vi "Calibration Table.vi"() -> ()   [LabVIEW 2015]
uses:
  Type/_RT Command.ctl
  Type/_File Type.ctl
  <vilib>/Utility/config.llb/Read Key (String).vi
  Configuration/_Global Configuration.vi
  <vilib>/Utility/config.llb/Write Key (String).vi
  <vilib>/Utility/file.llb/Read From Spreadsheet File (DBL).vi
  <vilib>/Utility/config.llb/NI_LVConfig.lvlib
panel:
  in  "Export":bool
  in  "Import":bool
  in  "TableFiles":path[](array[path])=[path "C:/Documents and Settings/MYANG/My Documents/Ion Sniffer/Build/Default Q1 Calibration.cal", path "C:/Documents and Settings/MYANG/My Documents/Ion Sniffer/Build/Default Q2 Calibration.cal", path "C:/Documents and Settings/MYANG/My Documents/Ion Sniffer/Build/Default Q1 Calibration.cal", path "C:/Documents and Settings/MYANG/My Documents/Ion Sniffer/Build/Default Q2 Calibration.cal", path "C:/Documents and Settings/MYANG/My Documents/Ion Sniffer/Build/Default Q1 Resolution.res", path "C:/Documents and Settings/MYANG/My Documents/Ion Sniffer/Build/Default Q2 Resolution.res", path "C:/Documents and Settings/MYANG/My Documents/Ion Sniffer/Build/Default Q1 Resolution.res", path "C:/Documents and Settings/MYANG/My Documents/Ion Sniffer/Build/Default Q2 Resolution.res", path "C:/Documents and Settings/MYANG/My Documents/Ion Sniffer/Build/Default Q1 Resolution.res", path "C:/Documents and Settings/MYANG/My Documents/Ion Sniffer/Build/Default Q2 Resolution.res", path "C:/Documents and Settings/MYANG/My Documents/Ion Sniffer/Build/Default Q1 Resolution.res", path "C:/Documents and Settings/MYANG/My Documents/Ion Sniffer/Build/Default Q2 Resolution.res", path "C:/Documents and Settings/MYANG/My Documents/Ion Sniffer/Build/Default Q1 Resolution.res", path "C:/Documents and Settings/MYANG/My Documents/Ion Sniffer/Build/Default Q2 Resolution.res", path "C:/Documents and Settings/MYANG/My Documents/Ion Sniffer/Build/Default Q1 Resolution.res", path "C:/Documents and Settings/MYANG/My Documents/Ion Sniffer/Build/Default Q2 Resolution.res"]
  in  "Measured Mass":dbl=50.0 caption="Measured Mass\n(amu)" min=0.0 format="%#.6g"
  in  "Reference Mass":dbl=50.0 caption="Reference Mass\n(amu)" min=0.0 format="%#.6g"
  in  "DAC Value":i32=8340 min=0 step=1
  in  "Download":bool
  in  "UITable":i32(listbox)
  in  "Table Type":u16(ring) items=["Q1 +ve Mass Calibration Table", "Q2 +ve Mass Calibration Table", "Q1 -ve Mass Calibration Table", "Q2 -ve Mass Calibration Table", "Q1 +ve High Resolution Table", "Q2 +ve High Resolution Table", "Q1 +ve Medium Resolution Table", "Q2 +ve Medium Resolution Table", "Q1 +ve Low Resolution Table", "Q2 +ve Low Resolution Table", "Q1 -ve High Resolution Table", "Q2 -ve High Resolution Table", "Q1 -ve Medium Resolution Table", "Q2 -ve Medium Resolution Table", "Q1 -ve Low Resolution Table", "Q2 -ve Low Resolution Table"]
  in  "Change":bool
  in  "Current Point #:":i32=1 min=1 step=1
  in  "Delete":bool
  in  "Insert":bool
  out "File Path:":path=path "C:/Documents and Settings/MYANG/My Documents/Ion Sniffer/Build/Default Q2 Resolution.res"
  in  "Save":bool
  in  "Load":bool
  out "Graph":cluster{"all rows":dbl[], "all rows":dbl[]}(graph)={"all rows"=[50.0, 130.0, 174.0, 195.0, 397.0, 510.0, 609.0, 906.0], "all rows"=[8340.0, 8620.0, 8730.0, 8825.0, 9480.0, 9830.0, 10230.0, 11000.0]} caption="Q1 Mass Calibration"
  out "# of Entries":i32=8
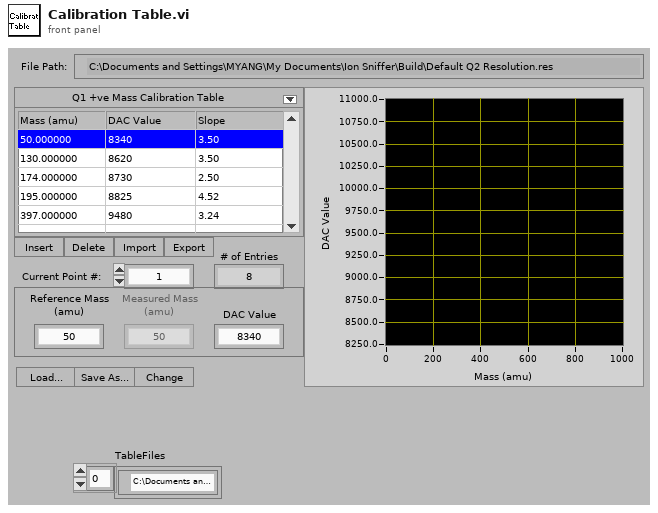
[diagram p1: front panel]
types:
  T1 = typedef "_RT Command.ctl" = enum16{"Start", "StartActualRun", "Stop", "Runtime Update", "Get Data", "Get Info", "Get Status", "Get Param", "Get Config", "Get Table", "Read ADC", "Set Oscillator", "Update Config", "Update Table", "Set All Pol", "Set Pol and DC", "Set Max Mass", "Toggle RP", "Toggle EL", "Set PIC", "Initialize Turbo", "Send Turbo Comm", "Close Turbo", "P1", "P2", "P3", "Send Serial", "Set LC Out", "Get LC In", "Read VAC", "Test Table", "Toggle Power", "Get Startup", "Set Startup", "Get ADC Table", "Set ADC Table", "Get Brief Status", "Get Detail Status", "Auxiliary Update", "Set CC Logics", "Set CC Input Logics", "Ignore Error"}
  T2 = typedef "_File Type.ctl" = enum16{"Configuration", "Old Configuration", "Calibration", "Resolution", "Diagnostic Method", "Old Method", "Acq Method", "Samp List"}
  T3 = enum32{"existing file", "new file", "new or existing file", "existing dir", "new dir", "new or existing dir", "existing file (use LLBs)", "new file (use LLBs)", "new or existing file (use LLBs)", "new or existing file or directory (use LLBs)"}
  T4 = typedef "NI_LVConfig.lvlib/Config Data RefNum.ctl" = refnum<k1>
  T5 = cluster{"Table":dbl[][], "Current Point #:":i32, "Update":bool, "TableFiles":path[]}
  T6 = typedef "_RT Configuration 2.ctl" = cluster{"Name":string, "Ch#":u8, "Min":dbl, "Max":dbl, "Def+":dbl, "Def-":dbl, "Offset":dbl, "Slope":dbl, "Type":u8, "Description":string, "SettleT":dbl}
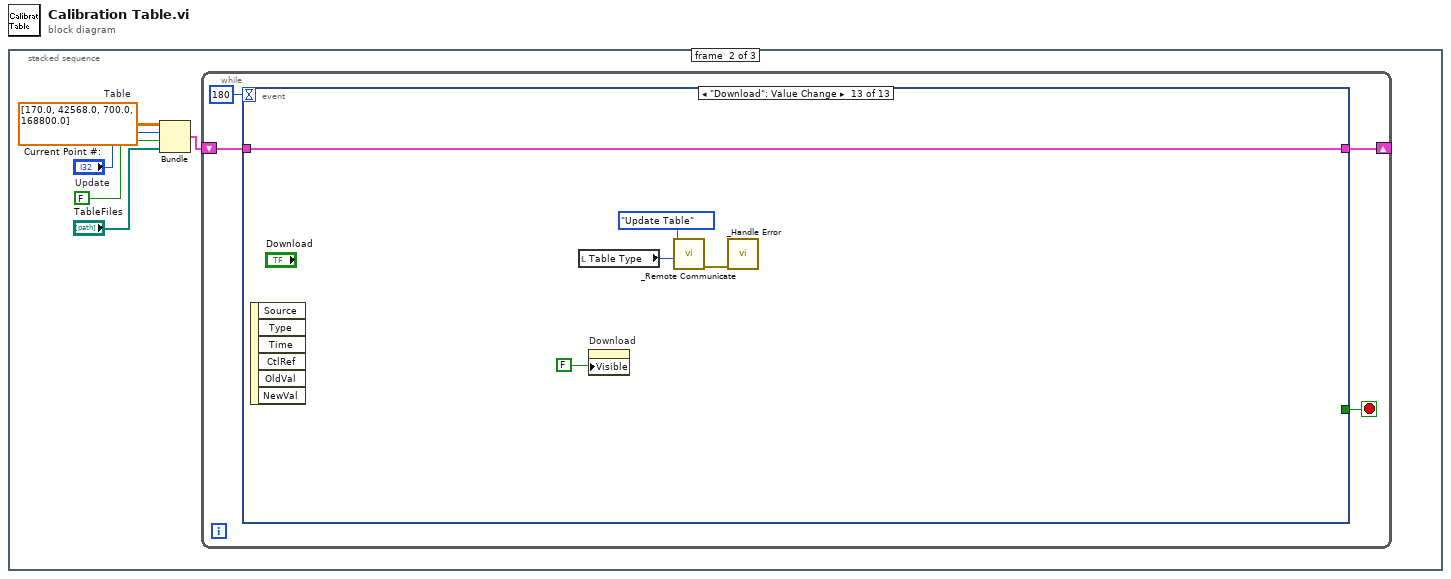
[diagram p0: block diagram]
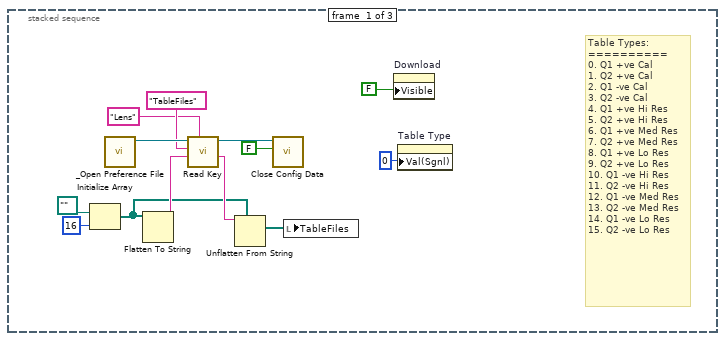
[diagram p2: hidden frame]
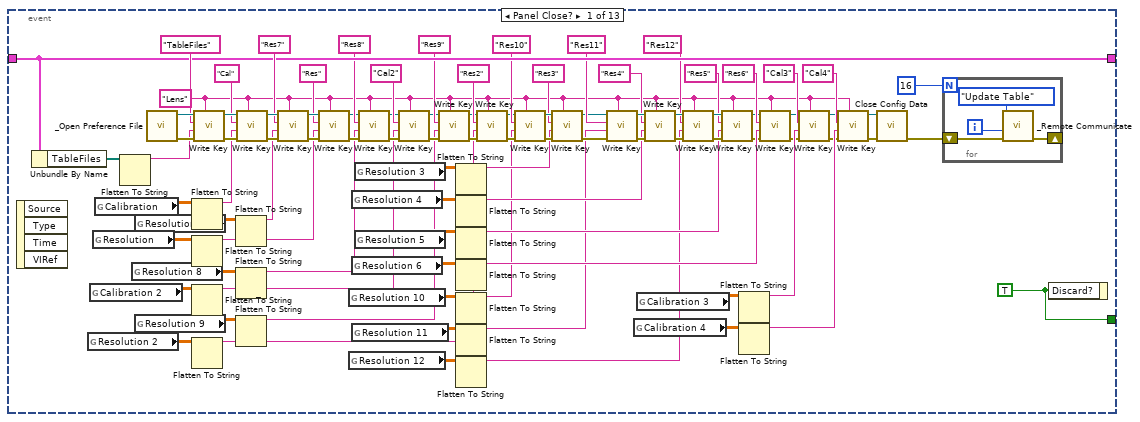
[diagram p3: hidden frame]
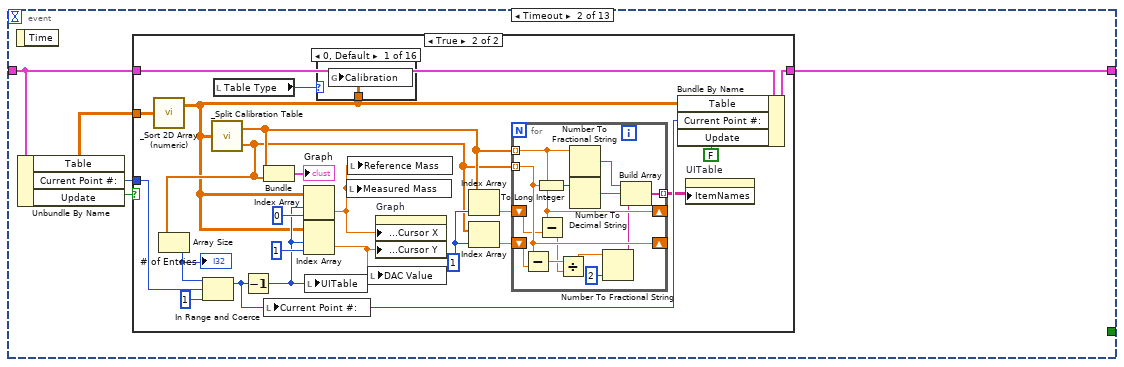
[diagram p4: hidden frame]
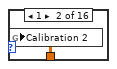
[diagram p6: hidden frame]
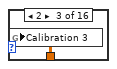
[diagram p7: hidden frame]
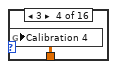
[diagram p8: hidden frame]
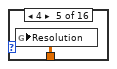
[diagram p9: hidden frame]
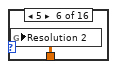
[diagram p10: hidden frame]
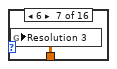
[diagram p11: hidden frame]
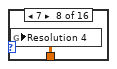
[diagram p12: hidden frame]
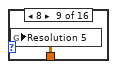
[diagram p13: hidden frame]
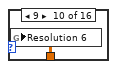
[diagram p14: hidden frame]
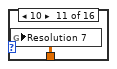
[diagram p15: hidden frame]
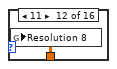
[diagram p16: hidden frame]
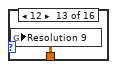
[diagram p17: hidden frame]
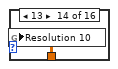
[diagram p18: hidden frame]
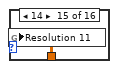
[diagram p19: hidden frame]
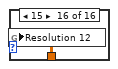
[diagram p20: hidden frame]
diagram:
  n1 = stacked-sequence {
    frame #0 {
      # "Table Types:\n==========\n0. Q1 +ve Cal\n1. Q2 +ve Cal\n2. Q1 -ve Cal\n3. Q2 -ve Cal\n4. Q1 +ve Hi Res\n5. Q2 +ve Hi Res\n6. Q1 +ve Med Res\n7. Q2 +ve Med Res\n8. Q1 +ve Lo Res\n9. Q2 +ve Lo Res\n10. Q1 -ve Hi Res\n11. Q2 -ve Hi Res\n12. Q1 -ve Med Res\n13. Q2 -ve Med Res\n14. Q1 -ve Lo Res\n15. Q2 -ve Lo Res"
      n2 = Initialize Array(path "", 16 ("dimension size")) -> (w2:path[])
      n3 = call "_Open Preference File.vi"() -> ("refnum"=w13:T4)  [unwired: 2 in, 5 out]
      n4 = Flatten To String(anything=w2) -> (data string=w7:string)  [unwired: 1 in, 4 out]
      n5 = call-poly <vilib>:"Read Key.vi"("section"="Lens", "default value"=w7, "key"="TableFiles" ("section"), "refnum"=w13) -> ("value"=w6:string, "refnum out"=w5:T4)  [unwired: 2 in, 4 out]
      n6 = Unflatten From String(type=w2, binary string=w6) -> (value=w1:path[])  [unwired: 1 in, 4 out]
      n7 = call <vilib>:"Close Config Data.vi"("write file if changed (T)"=FALSE ("write configuration file? (T)"), "refnum"=w5) -> ()  [unwired: 1 in, 9 out]
      n8 = local write "TableFiles"(w1) -> ()
      n9 = property on="Download" class="Bool"("Visible"=FALSE) -> ()  [unwired: 2 in, 2 out]
      n10 = property on="Table Type" class="Ring (strict)"("Val(Sgnl)"=u16 0 ("Value (Signaling)")) -> ()  [unwired: 2 in, 2 out]
    }
    frame #1 {
      w17 = FALSE  # Update
      w18 = dbl[][] [[170.0, 42568.0], [700.0, 168800.0]]  # Table
      n11 = Bundle("Table"=w18, "Current Point #:"="Current Point #:", "Update"=w17, "TableFiles"="TableFiles") -> (w16:T5)  [unwired: 1 out]
      n12 = while {
        shift-right: [w20] -> _
        shift-left: w16 -> [w21]
        stop <- w19 stop-if-true
        n13 = event shown="[12] \"Download\": Value Change" {
          selector: _ -> [_ _ _ _ _ _ _ _ _ _ _ _ _]
          dyn-events: _ -> [_ _ _ _ _ _ _ _ _ _ _ _ _]
          timeout: 180 -> [_ _ _ _ _ _ _ _ _ _ _ _ _]
          tunnel: w21 -> [w97 w121 w181 w238 w242 w246 w267 w287 w307 w333 w390 w416 w431]
          tunnel: [w97 w120 w185 w237 w241 w245 w266 w294 w307 w332 w389 w415 w431] -> w20
          tunnel: [w114 _ _ _ _ _ _ _ _ _ _ _ _] -> w19
          event Panel Close? {
            w51 = "Lens" ("section")
            w114 = TRUE ("Discard?")
            n14 = event-data() -> ()  [unwired: 5 out]
            n15 = Unbundle By Name(w97) -> ("TableFiles"=w44:path[])
            n16 = global read "_Global Configuration.vi" "Resolution 2"() -> (w84:dbl[][])
            n17 = global read "_Global Configuration.vi" "Calibration 2"() -> (w83:dbl[][])
            n18 = global read "_Global Configuration.vi" "Resolution"() -> (w99:dbl[][])
            n19 = global read "_Global Configuration.vi" "Calibration"() -> (w101:dbl[][])
            n20 = Flatten To String(anything=w44) -> (data string=w43:string)  [unwired: 1 in, 4 out]
            n21 = global read "_Global Configuration.vi" "Resolution 8"() -> (w38:dbl[][])
            n22 = global read "_Global Configuration.vi" "Resolution 7"() -> (w37:dbl[][])
            n23 = global read "_Global Configuration.vi" "Resolution 9"() -> (w39:dbl[][])
            n24 = call "_Open Preference File.vi"() -> ("error"=w110:errorcluster, "refnum"=w111:T4)  [unwired: 2 in, 4 out]
            n25 = Flatten To String(anything=w101) -> (data string=w100:string)  [unwired: 1 in, 4 out]
            n26 = Flatten To String(anything=w99) -> (data string=w98:string)  [unwired: 1 in, 4 out]
            n27 = Flatten To String(anything=w83) -> (data string=w82:string)  [unwired: 1 in, 4 out]
            n28 = Flatten To String(anything=w84) -> (data string=w81:string)  [unwired: 1 in, 4 out]
            n29 = call-poly <vilib>:"Write Key.vi"("section"=w51, "error in (no error)"=w110, "value"=w43, "key"="TableFiles" ("section"), "refnum"=w111) -> ("error out"=w113:errorcluster, "refnum out"=w112:T4)  [unwired: 1 in, 4 out]
            n30 = Flatten To String(anything=w37) -> (data string=w36:string)  [unwired: 1 in, 4 out]
            n31 = Flatten To String(anything=w38) -> (data string=w35:string)  [unwired: 1 in, 4 out]
            n32 = Flatten To String(anything=w39) -> (data string=w34:string)  [unwired: 1 in, 4 out]
            n33 = call-poly <vilib>:"Write Key.vi"("section"=w51, "error in (no error)"=w113, "value"=w100, "key"="Cal" ("section"), "refnum"=w112) -> ("error out"=w107:errorcluster, "refnum out"=w106:T4)  [unwired: 1 in, 4 out]
            n34 = call-poly <vilib>:"Write Key.vi"("section"=w51, "error in (no error)"=w107, "value"=w36, "key"="Res7" ("section"), "refnum"=w106) -> ("error out"=w108:errorcluster, "refnum out"=w109:T4)  [unwired: 1 in, 4 out]
            n35 = call-poly <vilib>:"Write Key.vi"("section"=w51, "error in (no error)"=w108, "value"=w98, "key"="Res" ("section"), "refnum"=w109) -> ("error out"=w86:errorcluster, "refnum out"=w85:T4)  [unwired: 1 in, 4 out]
            n36 = global read "_Global Configuration.vi" "Resolution 10"() -> (w33:dbl[][])
            n37 = global read "_Global Configuration.vi" "Resolution 12"() -> (w32:dbl[][])
            n38 = global read "_Global Configuration.vi" "Resolution 4"() -> (w59:dbl[][])
            n39 = global read "_Global Configuration.vi" "Resolution 6"() -> (w60:dbl[][])
            n40 = global read "_Global Configuration.vi" "Resolution 11"() -> (w31:dbl[][])
            n41 = global read "_Global Configuration.vi" "Resolution 3"() -> (w58:dbl[][])
            n42 = global read "_Global Configuration.vi" "Resolution 5"() -> (w61:dbl[][])
            n43 = call-poly <vilib>:"Write Key.vi"("section"=w51, "error in (no error)"=w86, "value"=w35, "key"="Res8" ("section"), "refnum"=w85) -> ("error out"=w87:errorcluster, "refnum out"=w88:T4)  [unwired: 1 in, 4 out]
            n44 = call-poly <vilib>:"Write Key.vi"("section"=w51, "error in (no error)"=w87, "value"=w82, "key"="Cal2" ("section"), "refnum"=w88) -> ("error out"=w91:errorcluster, "refnum out"=w92:T4)  [unwired: 1 in, 4 out]
            n45 = call-poly <vilib>:"Write Key.vi"("section"=w51, "error in (no error)"=w91, "value"=w34, "key"="Res9" ("section"), "refnum"=w92) -> ("error out"=w90:errorcluster, "refnum out"=w89:T4)  [unwired: 1 in, 4 out]
            n46 = Flatten To String(anything=w58) -> (data string=w57:string)  [unwired: 1 in, 4 out]
            n47 = Flatten To String(anything=w59) -> (data string=w56:string)  [unwired: 1 in, 4 out]
            n48 = Flatten To String(anything=w61) -> (data string=w55:string)  [unwired: 1 in, 4 out]
            n49 = Flatten To String(anything=w60) -> (data string=w54:string)  [unwired: 1 in, 4 out]
            n50 = Flatten To String(anything=w33) -> (data string=w30:string)  [unwired: 1 in, 4 out]
            n51 = Flatten To String(anything=w31) -> (data string=w29:string)  [unwired: 1 in, 4 out]
            n52 = Flatten To String(anything=w32) -> (data string=w28:string)  [unwired: 1 in, 4 out]
            n53 = call-poly <vilib>:"Write Key.vi"("section"=w51, "error in (no error)"=w90, "value"=w81, "key"="Res2" ("section"), "refnum"=w89) -> ("error out"=w75:errorcluster, "refnum out"=w76:T4)  [unwired: 1 in, 4 out]
            n54 = call-poly <vilib>:"Write Key.vi"("section"=w51, "error in (no error)"=w75, "value"=w30, "key"="Res10" ("section"), "refnum"=w76) -> ("error out"=w79:errorcluster, "refnum out"=w80:T4)  [unwired: 1 in, 4 out]
            n55 = call-poly <vilib>:"Write Key.vi"("section"=w51, "error in (no error)"=w79, "value"=w57, "key"="Res3" ("section"), "refnum"=w80) -> ("error out"=w63:errorcluster, "refnum out"=w62:T4)  [unwired: 1 in, 4 out]
            n56 = call-poly <vilib>:"Write Key.vi"("section"=w51, "error in (no error)"=w63, "value"=w29, "key"="Res11" ("section"), "refnum"=w62) -> ("error out"=w73:errorcluster, "refnum out"=w72:T4)  [unwired: 1 in, 4 out]
            n57 = global read "_Global Configuration.vi" "Calibration 4"() -> (w50:dbl[][])
            n58 = global read "_Global Configuration.vi" "Calibration 3"() -> (w49:dbl[][])
            n59 = call-poly <vilib>:"Write Key.vi"("section"=w51, "error in (no error)"=w73, "value"=w56, "key"="Res4" ("section"), "refnum"=w72) -> ("error out"=w69:errorcluster, "refnum out"=w68:T4)  [unwired: 1 in, 4 out]
            n60 = call-poly <vilib>:"Write Key.vi"("section"=w51, "error in (no error)"=w69, "value"=w28, "key"="Res12" ("section"), "refnum"=w68) -> ("error out"=w70:errorcluster, "refnum out"=w71:T4)  [unwired: 1 in, 4 out]
            n61 = call-poly <vilib>:"Write Key.vi"("section"=w51, "error in (no error)"=w70, "value"=w55, "key"="Res5" ("section"), "refnum"=w71) -> ("error out"=w27:errorcluster, "refnum out"=w42:T4)  [unwired: 1 in, 4 out]
            n62 = Flatten To String(anything=w49) -> (data string=w48:string)  [unwired: 1 in, 4 out]
            n63 = Flatten To String(anything=w50) -> (data string=w47:string)  [unwired: 1 in, 4 out]
            n64 = call-poly <vilib>:"Write Key.vi"("section"=w51, "error in (no error)"=w27, "value"=w54, "key"="Res6" ("section"), "refnum"=w42) -> ("error out"=w26:errorcluster, "refnum out"=w41:T4)  [unwired: 1 in, 4 out]
            n65 = call-poly <vilib>:"Write Key.vi"("section"=w51, "error in (no error)"=w26, "value"=w48, "key"="Cal3" ("section"), "refnum"=w41) -> ("error out"=w25:errorcluster, "refnum out"=w40:T4)  [unwired: 1 in, 4 out]
            n66 = call-poly <vilib>:"Write Key.vi"("section"=w51, "error in (no error)"=w25, "value"=w47, "key"="Cal4" ("section"), "refnum"=w40) -> ("error out"=w45:errorcluster, "refnum out"=w46:T4)  [unwired: 1 in, 4 out]
            n67 = call <vilib>:"Close Config Data.vi"("error in (no error)"=w45, "refnum"=w46) -> ("error out"=w24:errorcluster)  [unwired: 1 in, 8 out]
            n68 = for {
              N: 16 -> [_]
              shift-right: [w116] -> _
              shift-left: w24 -> [w117]
              i -> [w115]
              n69 = call "_Remote Communicate.vi"("error in (no error)"=w117, "DC Param"=w115, "Command"=_RT_Command."Update Table") -> ("error out"=w116:errorcluster)  [unwired: 3 in, 3 out]
            }
            n70 = event-data("Discard?"=w114) -> ()  [unwired: 1 in, 1 out]
          }
          event Timeout {
            n71 = event-data() -> ()  [unwired: 2 out]
            n72 = Unbundle By Name(w121) -> ("Table"=w119:dbl[][], "Current Point #:"=w122:i32, "Update"=w123:bool)
            n73 = case shown="True" w123 {
              tunnel: w119 -> [_ w141]
              tunnel: w122 -> [_ w143]
              tunnel: w121 -> [w124 w140]
              tunnel: [w124 w139] -> w120
              frame False {
              }
              frame True {
                w131 = 1 ("index")
                n74 = call "_Sort 2D Array (numeric).vi"("Unsorted 2D Array"=w141) -> ("Sorted 2D Array"=w126:dbl[][])  [unwired: 4 in, 1 out]
                n75 = call "_Split Calibration Table.vi"("Calibration"=w126) -> ("Mass"=w132:dbl[], "DAC"=w130:dbl[])
                n76 = Array Size(array=w130) -> (size(s)=w134:i32)
                "# of Entries" <- w134
                n77 = In Range and Coerce(upper limit=w134, x=w143, lower limit=1) -> (coerced(x)=w138:i32)  [unwired: 1 out]
                n78 = local read "Table Type"() -> (w127:u16)
                n79 = Decrement(x=w138) -> (x-1=w142:i32)
                n80 = Bundle("Mass"=w132, "DAC"=w130) -> (→"Graph":cluster{"Mass":dbl[], "DAC":dbl[]})  [unwired: 1 out]
                n81 = local write "Current Point #:"(w138) -> ()
                n82 = Index Array(array=w126, index (row)=w142, index (col)=0 ("Index")) -> (element=w135:dbl)
                n83 = Index Array(array=w126, index (row)=w142, index (col)=1 ("Index")) -> (element=w125:dbl)
                n84 = local write "UITable"(w142) -> ()
                n85 = case shown="0, Default" w127 {
                  tunnel: w126 -> [w147 w148 w149 w150 w151 w152 w153 w154 w155 w156 w157 w158 w159 w160 w161 w162]
                  frame 0, Default {
                    n86 = global write "_Global Configuration.vi" "Calibration"(w147) -> ()
                  }
                  frame 1 {
                    n87 = global write "_Global Configuration.vi" "Calibration 2"(w148) -> ()
                  }
                  frame 2 {
                    n88 = global write "_Global Configuration.vi" "Calibration 3"(w149) -> ()
                  }
                  frame 3 {
                    n89 = global write "_Global Configuration.vi" "Calibration 4"(w150) -> ()
                  }
                  frame 4 {
                    n90 = global write "_Global Configuration.vi" "Resolution"(w151) -> ()
                  }
                  frame 5 {
                    n91 = global write "_Global Configuration.vi" "Resolution 2"(w152) -> ()
                  }
                  frame 6 {
                    n92 = global write "_Global Configuration.vi" "Resolution 3"(w153) -> ()
                  }
                  frame 7 {
                    n93 = global write "_Global Configuration.vi" "Resolution 4"(w154) -> ()
                  }
                  frame 8 {
                    n94 = global write "_Global Configuration.vi" "Resolution 5"(w155) -> ()
                  }
                  frame 9 {
                    n95 = global write "_Global Configuration.vi" "Resolution 6"(w156) -> ()
                  }
                  frame 10 {
                    n96 = global write "_Global Configuration.vi" "Resolution 7"(w157) -> ()
                  }
                  frame 11 {
                    n97 = global write "_Global Configuration.vi" "Resolution 8"(w158) -> ()
                  }
                  frame 12 {
                    n98 = global write "_Global Configuration.vi" "Resolution 9"(w159) -> ()
                  }
                  frame 13 {
                    n99 = global write "_Global Configuration.vi" "Resolution 10"(w160) -> ()
                  }
                  frame 14 {
                    n100 = global write "_Global Configuration.vi" "Resolution 11"(w161) -> ()
                  }
                  frame 15 {
                    n101 = global write "_Global Configuration.vi" "Resolution 12"(w162) -> ()
                  }
                }
                n102 = local write "Measured Mass"(w135) -> ()
                n103 = local write "Reference Mass"(w135) -> ()
                n104 = local write "DAC Value"(w125) -> ()
                n105 = property on="Graph" class="XYGraph (strict)"("Cursor.Cursor Position:Cursor X"=w135, "Cursor.Cursor Position:Cursor Y"=w125) -> ()  [unwired: 2 in, 2 out]
                n106 = Index Array(array=w132, index=w131) -> (element=w129:dbl)
                n107 = Index Array(array=w130, index=w131) -> (element=w128:dbl)
                n108 = for {
                  tunnel: [w172] -> w133 mode=indexing
                  tunnel: w132 -> [w169] mode=indexing
                  tunnel: w130 -> [w171] mode=indexing
                  shift-right: [w169] -> _
                  shift-left: w129 -> [w168]
                  shift-right: [w171] -> _
                  shift-left: w128 -> [w170]
                  n109 = Subtract(x=w171, y=w170) -> (x-y=w167:dbl)
                  n110 = To Long Integer(number=w171) -> (32bit integer=w175:i32)
                  n111 = Subtract(x=w169, y=w168) -> (x-y=w166:dbl)
                  n112 = Divide(x=w167, y=w166) -> (x/y=w165:dbl)
                  n113 = Number To Fractional String(number=w169) -> (F-format string=w174:string)  [unwired: 3 out]
                  n114 = Number To Decimal String(number=w175) -> (decimal integer string=w173:string)  [unwired: 1 out]
                  n115 = Number To Fractional String(number=w165, precision (6)=i16 2) -> (F-format string=w163:string)  [unwired: 2 out]
                  n116 = Build Array(w174, w173, w163) -> (w172:string[])
                }
                n117 = Bundle By Name(cluster=w140, "Table"=w126, "Current Point #:"=w138, "Update"=FALSE) -> (w139:T5)
                n118 = property on="UITable" class="MCListbox (strict)"("ItemNames"=w133) -> ()  [unwired: 2 in, 2 out]
              }
            }
          }
          event "Table Type": Value Change {
            n119 = event-data() -> ("NewVal"=w177:u16)  [unwired: 1 out]
            n120 = Unbundle By Name(w181) -> ("TableFiles"=w178:path[])
            n121 = Index Array(array=w178, index=w177) -> (element=w176:path)
            n122 = local write "File Path:"(w176) -> ()
            n123 = case shown="0, Default" w177 {
              tunnel: [w188 w191 w194 w197 w200 w203 w206 w209 w212 w215 w218 w221 w224 w227 w230 w233] -> w182
              tunnel: [u8 0 ("Disabled") u8 0 ("Disabled") u8 0 ("Disabled") u8 0 ("Disabled") u8 2 ("Disabled") u8 2 ("Disabled") u8 2 ("Disabled") u8 2 ("Disabled") u8 2 ("Disabled") u8 2 ("Disabled") u8 2 ("Disabled") u8 2 ("Disabled") u8 2 ("Disabled") u8 2 ("Disabled") u8 2 ("Disabled") u8 2 ("Disabled")] -> w180
              tunnel: [u8 2 ("Disabled") u8 2 ("Disabled") u8 2 ("Disabled") u8 2 ("Disabled") u8 0 ("Disabled") u8 0 ("Disabled") u8 0 ("Disabled") u8 0 ("Disabled") u8 0 ("Disabled") u8 0 ("Disabled") u8 0 ("Disabled") u8 0 ("Disabled") u8 0 ("Disabled") u8 0 ("Disabled") u8 0 ("Disabled") u8 0 ("Disabled")] -> w179
              frame 0, Default {
                # "Q1 +ve Calibration"
                n124 = global read "_Global Configuration.vi" "Calibration"() -> (w188:dbl[][])
              }
              frame 1 {
                # "Q2 +ve Calibration"
                n125 = global read "_Global Configuration.vi" "Calibration 2"() -> (w191:dbl[][])
              }
              frame 2 {
                # "Q1 -ve Calibration"
                n126 = global read "_Global Configuration.vi" "Calibration 3"() -> (w194:dbl[][])
              }
              frame 3 {
                # "Q2 -ve Calibration"
                n127 = global read "_Global Configuration.vi" "Calibration 4"() -> (w197:dbl[][])
              }
              frame 4 {
                # "Q1 +ve Hi Resolution"
                n128 = global read "_Global Configuration.vi" "Resolution"() -> (w200:dbl[][])
              }
              frame 5 {
                # "Q2 +ve Hi Resolution"
                n129 = global read "_Global Configuration.vi" "Resolution 2"() -> (w203:dbl[][])
              }
              frame 6 {
                # "Q1 +ve Med Resolution"
                n130 = global read "_Global Configuration.vi" "Resolution 3"() -> (w206:dbl[][])
              }
              frame 7 {
                # "Q2 +ve Med Resolution"
                n131 = global read "_Global Configuration.vi" "Resolution 4"() -> (w209:dbl[][])
              }
              frame 8 {
                # "Q1 +ve Low Resolution"
                n132 = global read "_Global Configuration.vi" "Resolution 5"() -> (w212:dbl[][])
              }
              frame 9 {
                # "Q2 +ve Low Resolution"
                n133 = global read "_Global Configuration.vi" "Resolution 6"() -> (w215:dbl[][])
              }
              frame 10 {
                # "Q1 -ve Hi Resolution"
                n134 = global read "_Global Configuration.vi" "Resolution 7"() -> (w218:dbl[][])
              }
              frame 11 {
                # "Q2 -ve Hi Resolution"
                n135 = global read "_Global Configuration.vi" "Resolution 8"() -> (w221:dbl[][])
              }
              frame 12 {
                # "Q1 -ve Med Resolution"
                n136 = global read "_Global Configuration.vi" "Resolution 9"() -> (w224:dbl[][])
              }
              frame 13 {
                # "Q2 -ve Med Resolution"
                n137 = global read "_Global Configuration.vi" "Resolution 10"() -> (w227:dbl[][])
              }
              frame 14 {
                # "Q1 -ve Low Resolution"
                n138 = global read "_Global Configuration.vi" "Resolution 11"() -> (w230:dbl[][])
              }
              frame 15 {
                # "Q2 -ve Low Resolution"
                n139 = global read "_Global Configuration.vi" "Resolution 12"() -> (w233:dbl[][])
              }
            }
            n140 = property on="Measured Mass" class="DigNum (strict)"("Disabled"=w180) -> ()  [unwired: 2 in, 2 out]
            n141 = property on="DAC Value" class="DigNum (strict)"("Disabled"=w179) -> ()  [unwired: 2 in, 2 out]
            n142 = Bundle By Name(cluster=w181, "Table"=w182, "Current Point #:"=1, "Update"=TRUE) -> (w185:T5)
          }
          event "UITable": Value Change {
            n143 = event-data() -> ("NewVal"=w236:i32)  [unwired: 1 out]
            n144 = Increment(x=w236) -> (x+1=w234:i32)
            n145 = Bundle By Name(cluster=w238, "Current Point #:"=w234, "Update"=TRUE) -> (w237:T5)
          }
          event "Current Point #:": Value Change {
            n146 = event-data() -> ("NewVal"=w239:i32)  [unwired: 1 out]
            n147 = Bundle By Name(cluster=w242, "Current Point #:"=w239, "Update"=TRUE) -> (w241:T5)
          }
          event "Save": Value Change {
            n148 = event-data() -> ()  [unwired: 7 out]
            n149 = Unbundle By Name(w246) -> ("Table"=w247:dbl[][], "TableFiles"=w244:path[])
            n150 = case shown="4..15" "Table Type" {
              tunnel: [_File_Type."Calibration" ("File Type (config)") _File_Type."Resolution" ("File Type (config)")] -> w251
              frame 0, Default {
              }
              frame 4..15 {
              }
            }
            n151 = local read "File Path:"() -> (w252:path)
            n152 = call "_Save Config File.vi"("File Type (config)"=w251, "Cal/Res"=w247, "start path  (Not A Path)"=w252) -> ("error"=w250:bool, "new file path"=w249:path)  [unwired: 5 in, 2 out]
            n153 = case shown="False" w250 {
              tunnel: w249 -> [w254 _]
              tunnel: "Table Type" -> [w255 _]
              tunnel: w246 -> [w258 w259]
              tunnel: [w257 w259] -> w245
              tunnel: w244 -> [w256 _]
              frame False {
                n154 = Replace Array Subset(array=w256, new element=w254, index=w255) -> (w253:path[])
                n155 = Bundle By Name(cluster=w258, "TableFiles"=w253) -> (w257:T5)
                "File Path:" <- w254
              }
              frame True {
              }
            }
            n156 = local write "Save"(FALSE ("Save")) -> ()
          }
          event "Load": Value Change {
            n157 = event-data() -> ()  [unwired: 7 out]
            n158 = local read "Table Type"() -> (w263:u16)
            n159 = case shown="4..15" w263 {
              tunnel: [_File_Type."Calibration" ("File Type (config)") _File_Type."Resolution" ("File Type (config)")] -> w262
              frame 0, Default {
              }
              frame 4..15 {
              }
            }
            n160 = local read "File Path:"() -> (w269:path)
            n161 = call "_Read Config File.vi"("File Type (config)"=w262, "start path  (Not A Path)"=w269) -> ("error"=w268:bool, "Cal/Res"=w264:dbl[][], "new file path"=w265:path)  [unwired: 1 in, 6 out]
            n162 = case shown="False" w268 {
              tunnel: w267 -> [w276 w282]
              tunnel: [w279 w282] -> w266
              tunnel: w265 -> [w273 _]
              tunnel: w264 -> [w278 _]
              tunnel: w263 -> [w274 _]
              frame False {
                n163 = local write "File Path:"(w273) -> ()
                n164 = property on="Download" class="Bool"("Visible"=TRUE) -> ()  [unwired: 2 in, 2 out]
                n165 = Unbundle By Name(w276) -> ("TableFiles"=w275:path[])
                n166 = Replace Array Subset(array=w275, new element=w273, index=w274) -> (w272:path[])
                n167 = Bundle By Name(cluster=w276, "TableFiles"=w272, "Table"=w278, "Current Point #:"=1, "Update"=TRUE) -> (w279:T5)
              }
              frame True {
              }
            }
          }
          event "Import": Value Change {
            n168 = event-data() -> ()  [unwired: 2 out]
            n169 = Unbundle By Name(w287) -> ("TableFiles"=w286:path[])
            n170 = Index Array(array=w286) -> (element=w285:path)  [unwired: 1 in]
            n171 = call "_Get File.vi"("For Write (T)"=FALSE, "select mode (new or existing)"=T3."existing file", "extension (isd)"="*.txt" ("pattern (all files)"), "prompt"="Please select a table export file.", "Start Path"=w285) -> ("Seleted File"=w283:path, "Exists"=w288:bool, "Succeeded"=w289:bool)  [unwired: 1 in, 1 out]
            n172 = And(x=w289, y=w288) -> (x .and. y?=w284:bool)
            n173 = case shown="True" w284 {
              tunnel: w287 -> [w295 w301]
              tunnel: [w295 w303] -> w294
              tunnel: w283 -> [_ w300]
              frame False {
              }
              frame True {
                n174 = call-poly <vilib>:"Read From Spreadsheet File.vi"("file path (dialog if empty)"=w300) -> ("all rows"=w297:dbl[][])  [unwired: 3 in, 7 out]
                n175 = Delete From Array(array=w297, length=1, index (row)=0) -> (array with subset deleted=w296:dbl[][])  [unwired: 1 in, 1 out]
                n176 = Bundle By Name(cluster=w301, "Table"=w296, "Current Point #:"=1, "Update"=TRUE) -> (w303:T5)
                n177 = property on="Download" class="Bool"("Visible"=TRUE) -> ()  [unwired: 2 in, 2 out]
              }
            }
          }
          event "Export": Value Change {
            n178 = event-data() -> ()  [unwired: 2 out]
            n179 = Unbundle By Name(w307) -> ("Table"=w308:dbl[][], "TableFiles"=w312:path[])
            n180 = Index Array(array=w312) -> (element=w311:path)  [unwired: 1 in]
            n181 = call "_Get File.vi"("For Write (T)"=TRUE, "select mode (new or existing)"=T3."new or existing file", "default name"="My Table", "extension (isd)"="*.txt" ("pattern (all files)"), "prompt"="Please enter a table export file name.", "Start Path"=w311) -> ("Seleted File"=w310:path, "Succeeded"=w309:bool)  [unwired: 2 out]
            n182 = case shown="True" w309 {
              tunnel: w310 -> [_ w321]
              tunnel: w308 -> [_ w320]
              frame False {
              }
              frame True {
                n183 = Number To Fractional String(number=w320) -> (F-format string=w319:string[][])  [unwired: 3 out]
                n184 = Build Array (concatenate)(string[] ["Mass (amu)", "DAC"], w319) -> (w317:string[][])
                n185 = call "_Export Table To Text File.vi"("2D data"=w317, "file path (dialog if empty)"=w321) -> ()  [unwired: 4 in, 3 out]
              }
            }
          }
          event "Change": Value Change {
            n186 = event-data() -> ()  [unwired: 2 out]
            n187 = Unbundle By Name(w333) -> ("Table"=w334:dbl[][])
            n188 = local read "Table Type"() -> (w328:u16)
            n189 = To Double Precision Float(number="DAC Value") -> (double precision float=w326:dbl)
            n190 = property on="Download" class="Bool"("Visible"=TRUE) -> ()  [unwired: 2 in, 2 out]
            n191 = case shown="0, Default" w328 {
              tunnel: w326 -> [w344 w351 w353 w360]
              tunnel: [w344 w350 w353 w359] -> w325
              tunnel: [u8 1 ("Channel #") u8 1 ("Channel #") u8 2 ("Channel #") u8 2 ("Channel #")] -> w323
              frame 0, Default {
                # "Q1 Cal"
              }
              frame 4, 6, 8, 10, 12, 14 {
                # "Q1 Res"
                n192 = call "_Get Lens Configuration.vi"("Channel #"=u8 7) -> ("Lens Configuration"=w348:T6)  [unwired: 1 in, 5 out]
                n193 = Unbundle By Name(w348) -> ("Max"=w347:dbl, "Min"=w346:dbl)
                n194 = In Range and Coerce(upper limit=w347, x=w351, lower limit=w346) -> (coerced(x)=w350:dbl)  [unwired: 1 out]
              }
              frame 1, 3 {
                # "Q2 Cal"
              }
              frame 5, 7, 9, 11, 13, 15 {
                # "Q2 Res"
                n195 = call "_Get Lens Configuration.vi"("Channel #"=u8 9) -> ("Lens Configuration"=w357:T6)  [unwired: 1 in, 5 out]
                n196 = Unbundle By Name(w357) -> ("Max"=w356:dbl, "Min"=w355:dbl)
                n197 = In Range and Coerce(upper limit=w356, x=w360, lower limit=w355) -> (coerced(x)=w359:dbl)  [unwired: 1 out]
              }
            }
            n198 = call "_Get Lens Configuration.vi"("Channel #"=w323) -> ("Lens Configuration"=w324:T6)  [unwired: 1 in, 5 out]
            n199 = Unbundle By Name(w324) -> ("Max"=w342:dbl, "Min"=w341:dbl)
            n200 = In Range and Coerce(upper limit=w342, x="Reference Mass", lower limit=w341) -> (coerced(x)=w322:dbl)  [unwired: 1 out]
            n201 = Equal?(x=w322, y="Measured Mass") -> (x = y?=w338:bool)
            n202 = case shown="False" w338 {
              tunnel: "Measured Mass" -> [w364 _]
              tunnel: w322 -> [w369 _]
              tunnel: w334 -> [w368 _]
              tunnel: [w367 w385] -> w339
              tunnel: w325 -> [w361 w385]
              frame False {
                n203 = property on="Graph" class="XYGraph (strict)"() -> ("Cursor.Cursor Y"=w362:dbl, "Cursor.Cursor Position:Cursor X"=w363:dbl)  [unwired: 2 in, 2 out]
                n204 = Not Equal?(x=w363, y=w364) -> (x != y?=w365:bool)
                n205 = Greater Than 0?(x=w364) -> (x > 0?=w366:bool)
                n206 = And(x=w365, y=w366) -> (x .and. y?=w370:bool)
                n207 = case shown="False" w370 {
                  tunnel: w369 -> [_ w379]
                  tunnel: w364 -> [w373 _]
                  tunnel: w368 -> [w372 w380]
                  tunnel: [w371 w378] -> w367
                  tunnel: w362 -> [_ w377]
                  tunnel: w361 -> [_ w375]
                  frame True {
                    # "measure mass\nchanged"
                    n208 = call "_Convert Mass to DAC.vi"("Calibration Table"=w372, "Mass"=w373) -> ("DAC Value"=w371:dbl)  [unwired: 2 in, 3 out]
                  }
                  frame False {
                    # "reference mass changed"
                    n209 = Round To Nearest(number=w377) -> (nearest integer value=w374:dbl)
                    n210 = Equal?(x=w375, y=w374) -> (x = y?=w376:bool)
                    n211 = case shown="True" w376 {
                      tunnel: w380 -> [_ w384]
                      tunnel: w379 -> [_ w383]
                      tunnel: [w381 w382] -> w378
                      tunnel: w375 -> [w381 _]
                      frame False {
                      }
                      frame True {
                        n212 = call "_Convert Mass to DAC.vi"("Calibration Table"=w384, "Mass"=w383) -> ("DAC Value"=w382:dbl)  [unwired: 2 in, 3 out]
                      }
                    }
                  }
                }
              }
              frame True {
                # "DAC value changed"
              }
            }
            n213 = Build Array(w322, w339) -> (w340:dbl[])
            n214 = Replace Array Subset(array=w334, new element=w340, index (row)="UITable") -> (w330:dbl[][])  [unwired: 1 in]
            n215 = Bundle By Name(cluster=w333, "Update"=TRUE, "Table"=w330) -> (w332:T5)
          }
          event "Insert": Value Change {
            n216 = event-data() -> ()  [unwired: 7 out]
            n217 = local read "# of Entries"() -> (w388:i32)
            n218 = Greater?(x=w388, y=23) -> (0:w386:bool)
            n219 = case shown="False" w386 {
              tunnel: w390 -> [w394 w410]
              tunnel: [w393 w410] -> w389
              frame False {
                w404 = 0 ("disabled index (col)")
                n220 = local read "UITable"() -> (w396:i32)
                n221 = Unbundle By Name(w394) -> ("Table"=w397:dbl[][])
                n222 = Max & Min(x=1, y=w396) -> (max(x,y)=w398:i32)  [unwired: 1 out]
                n223 = Decrement(x=w398) -> (x-1=w405:i32)
                n224 = Index Array(array=w397, index (row) #1=w398, index (col) #1=w404, index (row) #2=w405, index (col) #2=w404) -> (element #1=w403:dbl, element #2=w402:dbl)
                n225 = Add(x=w403, y=w402) -> (x+y=w401:dbl)
                n226 = Divide(x=w401, y=2.0) -> (x/y=w408:dbl)
                n227 = call "_Convert Mass to DAC.vi"("Calibration Table"=w397, "Mass"=w408) -> ("DAC Value"=w407:dbl)  [unwired: 2 in, 3 out]
                n228 = Build Array(w408, w407) -> (w406:dbl[])
                n229 = property on="Download" class="Bool"("Visible"=TRUE) -> ()  [unwired: 2 in, 2 out]
                n230 = Insert Into Array(array=w397, index (row)=w396, new element=w406) -> (w392:dbl[][])  [unwired: 1 in]
                n231 = Bundle By Name(cluster=w394, "Update"=TRUE, "Table"=w392) -> (w393:T5)
              }
              frame True {
                n232 = One Button Dialog(message="You are not allow to add more than 23 entries in the table due to hardware limitation.") -> ()  [unwired: 2 out]
              }
            }
          }
          event "Delete": Value Change {
            n233 = event-data() -> ()  [unwired: 7 out]
            n234 = local read "# of Entries"() -> (w413:i32)
            n235 = Unbundle By Name(w416) -> ("Table"=w411:dbl[][])
            n236 = Greater?(x=w413, y=2) -> (0:w414:bool)
            n237 = case shown="True" w414 {
              tunnel: w416 -> [w417 w425]
              tunnel: [w417 w424] -> w415
              tunnel: w411 -> [_ w422]
              frame False {
                n238 = One Button Dialog(message="You are not allow to delete the last two entries in the table.") -> ()  [unwired: 2 out]
              }
              frame True {
                n239 = local read "UITable"() -> (w421:i32)
                n240 = Delete From Array(array=w422, length=1, index (row)=w421) -> (array with subset deleted=w420:dbl[][])  [unwired: 1 in, 1 out]
                n241 = property on="Download" class="Bool"("Visible"=TRUE) -> ()  [unwired: 2 in, 2 out]
                n242 = Bundle By Name(cluster=w425, "Update"=TRUE, "Table"=w420) -> (w424:T5)
              }
            }
          }
          event "Download": Value Change {
            n243 = event-data() -> ()  [unwired: 7 out]
            n244 = local read "Table Type"() -> (w427:u16)
            n245 = property on="Download" class="Bool"("Visible"=FALSE) -> ()  [unwired: 2 in, 2 out]
            n246 = call "_Remote Communicate.vi"("DC Param"=w427, "Command"=_RT_Command."Update Table") -> ("error out"=w429:errorcluster)  [unwired: 4 in, 3 out]
            n247 = call "_Handle Error.vi"("error in (no error)"=w429) -> ()  [unwired: 2 in, 5 out]
          }
        }
      }
    }
    frame #2 {
      n248 = property class="VI"("Front Panel.Open"=FALSE ("Front Panel Window:Open")) -> ()  [unwired: 2 in, 2 out]
    }
  }
